vi "Wire Event Reg Through Case Structure.vi"(8 "error in (no error)":errorcluster, 11 "JKI SM in":refnum<class "JKI SM.lvclass">) -> (0 "error out":errorcluster, 3 "JKI SM out":refnum<class "JKI SM.lvclass">)   [LabVIEW 2020, in "JKI State Machine API.lvlib" / "JKI SM.lvclass"]
uses:
  JKI SM.lvclass
  JKI SM.lvclass/JKI SM.ctl
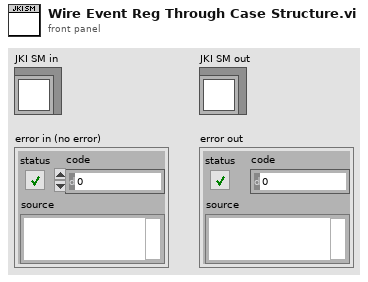
[diagram p1: front panel]
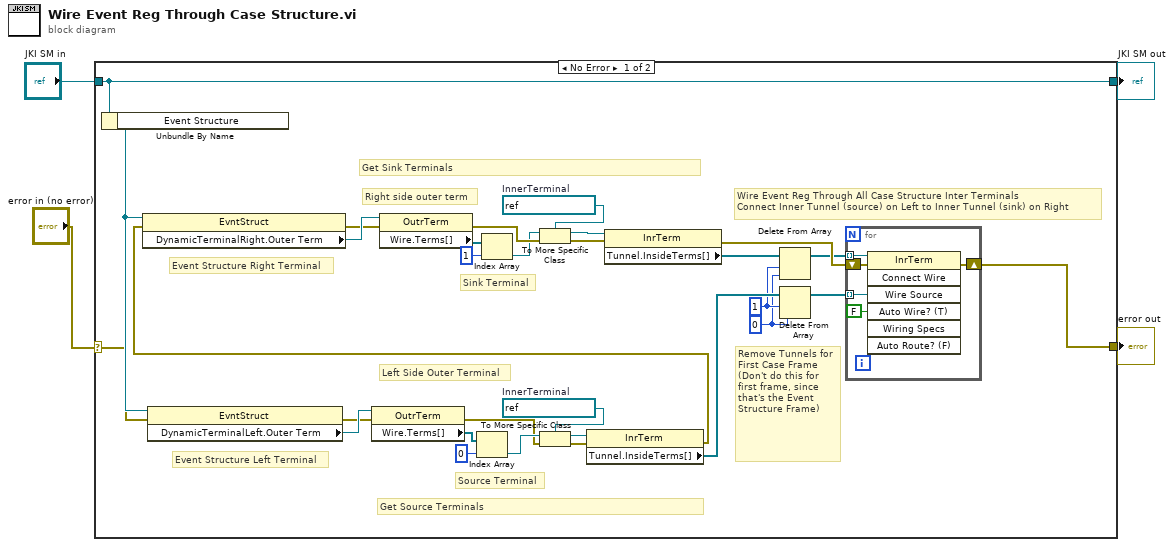
[diagram p0: block diagram]
diagram:
  n1 = case shown="No Error" "error in (no error)" {
    selector: "error in (no error)" -> [w7 w40]
    tunnel: [w21 w40] -> w1
    tunnel: "JKI SM in" -> [w5 w41]
    tunnel: [w5 w41] -> w4
    frame No Error {
      w13 = 0 ("index")
      w14 = 1 ("length")
      w26 = refnum<vi> refnum  # InnerTerminal
      w32 = refnum<vi> refnum  # InnerTerminal
      # "Event Structure Right Terminal"
      # "Event Structure Left Terminal"
      # "Get Sink Terminals"
      # "Get Source Terminals"
      # "Remove Tunnels for First Case Frame\n(Don't do this for first frame, since that's the Event Structure Frame)"
      # "Wire Event Reg Through All Case Structure Inter Terminals\nConnect Inner Tunnel (source) on Left to Inner Tunnel (sink) on Right"
      # "Left Side Outer Terminal"
      # "Right side outer term"
      # "Source Terminal"
      # "Sink Terminal"
      n2 = Unbundle By Name(w5) -> ("Event Structure"=w8:refnum<vi>)
      n3 = property class="EvntStruct"(reference=w8, error in=w7) -> (error out=w6:errorcluster, "DynamicTerminalLeft.Outer Term"=w9:refnum<vi>)  [unwired: 1 out]
      n4 = property class="OutrTerm"(reference=w9, error in=w6) -> (error out=w20:errorcluster, "Wire.Terms[]"=w27:refnum<vi>[])  [unwired: 1 out]
      n5 = Index Array(array=w27, index=0) -> (element=w25:refnum<vi>)
      n6 = To More Specific Class(target class=w26, reference=w25, error in=w20) -> (specific class reference=w24:refnum<vi>, error out=w19:errorcluster)
      n7 = property class="InrTerm"(reference=w24, error in=w19) -> (error out=w11:errorcluster, "Tunnel.InsideTerms[]"=w18:refnum<vi>[])  [unwired: 1 out]
      n8 = property class="EvntStruct"(reference=w8, error in=w11) -> (error out=w10:errorcluster, "DynamicTerminalRight.Outer Term"=w12:refnum<vi>)  [unwired: 1 out]
      n9 = property class="OutrTerm"(reference=w12, error in=w10) -> (error out=w31:errorcluster, "Wire.Terms[]"=w34:refnum<vi>[])  [unwired: 1 out]
      n10 = Index Array(array=w34, index=1) -> (element=w22:refnum<vi>)
      n11 = To More Specific Class(target class=w32, reference=w22, error in=w31) -> (specific class reference=w30:refnum<vi>, error out=w29:errorcluster)
      n12 = property class="InrTerm"(reference=w30, error in=w29) -> (error out=w23:errorcluster, "Tunnel.InsideTerms[]"=w16:refnum<vi>[])  [unwired: 1 out]
      n13 = Delete From Array(array=w16, length=w14, index=w13) -> (array with subset deleted=w15:refnum<vi>[])  [unwired: 1 out]
      n14 = Delete From Array(array=w18, length=w14, index=w13) -> (array with subset deleted=w17:refnum<vi>[])  [unwired: 1 out]
      n15 = for {
        tunnel: w15 -> [w39] mode=indexing
        tunnel: w17 -> [w38] mode=indexing
        shift-right: [w36] -> w21
        shift-left: w23 -> [w35]
        n16 = invoke class="InrTerm" method="Connect Wire"(reference=w39, error in=w35, "Wire Source"=w38, "Auto Wire? (T)"=FALSE) -> (error out=w36:errorcluster)  [unwired: 3 in, 6 out]
      }
    }
    frame Error {
    }
  }
  "JKI SM out" <- w4
  "error out" <- w1
